vi "image_data_to_double_precision.vi"(1 "Data In":cluster{"X":i32, "Y":i32}[][](array[cluster])) -> (0 "Data Out":cluster{"X":dbl, "Y":dbl}[][](array[cluster]))   [LabVIEW 2017]
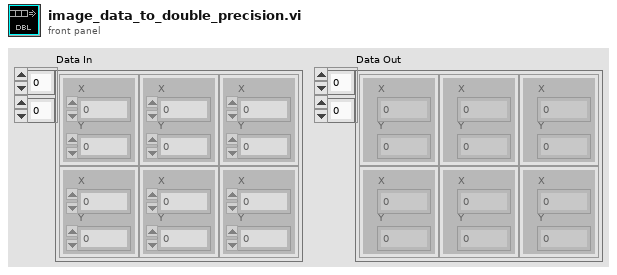
[diagram p1: front panel]
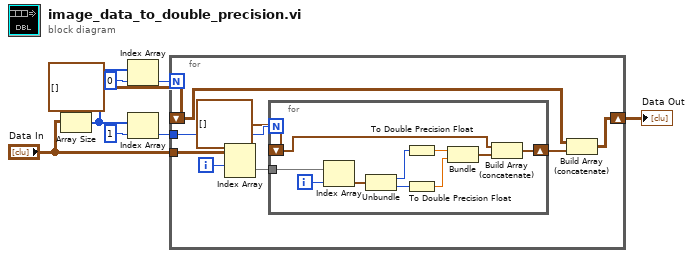
[diagram p0: block diagram]
diagram:
  n1 = Array Size(array="Data In") -> (size(s)=w4:i32[])
  n2 = Index Array(array=w4, index=0) -> (element=w7:i32)
  n3 = Index Array(array=w4, index=1) -> (element=w3:i32)
  n4 = for {
    N: w7 -> [_]
    tunnel: "Data In" -> [w16]
    tunnel: w3 -> [w14]
    shift-right: [w10] -> w2
    shift-left: cluster{dbl, dbl}[][] [] -> [w12]
    i -> [w15]
    n5 = Index Array(array=w16, index (row)=w15) -> (element=w13:cluster{"X":i32, "Y":i32}[])  [unwired: 1 in]
    n6 = for {
      N: w14 -> [_]
      shift-right: [w25] -> w11
      shift-left: cluster{dbl, dbl}[] [] -> [w26]
      tunnel: w13 -> [w24]
      i -> [w23]
      n7 = Index Array(array=w24, index=w23) -> (element=w22:cluster{"X":i32, "Y":i32})
      n8 = Unbundle(w22) -> ("X"=w21:i32, "Y"=w18:i32)
      n9 = To Double Precision Float(number=w21) -> (double precision float=w19:dbl)
      n10 = To Double Precision Float(number=w18) -> (double precision float=w20:dbl)
      n11 = Bundle(w19, w20) -> (w17:cluster{dbl, dbl})  [unwired: 1 in]
      n12 = Build Array (concatenate)(w26, w17) -> (w25:cluster{dbl, dbl}[])
    }
    n13 = Build Array (concatenate)(w12, w11) -> (w10:cluster{dbl, dbl}[][])
  }
  "Data Out" <- w2
